vi "Query.vi"(8 "error in (no error)":errorcluster, 10 "command":string, 11 "Toolbox in":refnum<class "Toolbox.lvclass">) -> (0 "error out":errorcluster, 2 "responses":string[](array[string]), 3 "Toolbox out":refnum<class "Toolbox.lvclass">)   [LabVIEW 2014, in "Driver_interaction.lvlib" / "Toolbox.lvclass"]
uses:
  Toolbox.lvclass
  Toolbox.lvclass/Toolbox.ctl
  _Driver_interaction/_Driver_interaction.lvclass
  Vendor/lib 2p0/FTS 2p0.lvlib
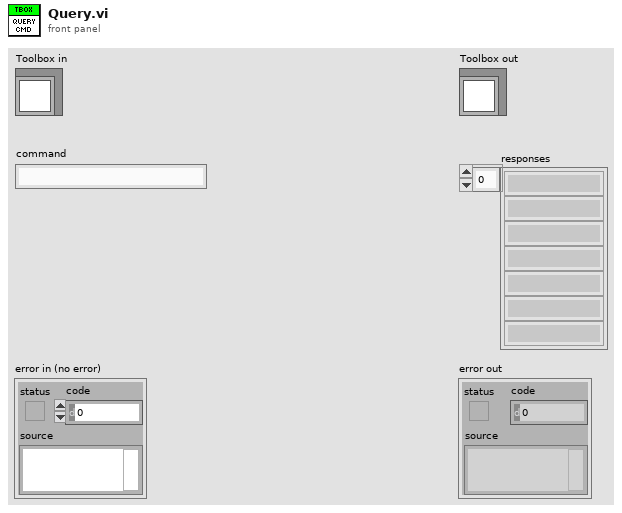
[diagram p1: front panel]
types:
  T1 = typedef "Driver_interaction.lvlib/Toolbox.lvclass/Toolbox_session.ctl" = cluster{"client handle":T2, "URL out":string, "universe_id":i32, "devices_id":i32[]}
  T2 = typedef "LabVIEWHTTPClient.lvlib/ClientHandle.ctl" = refnum<k1>
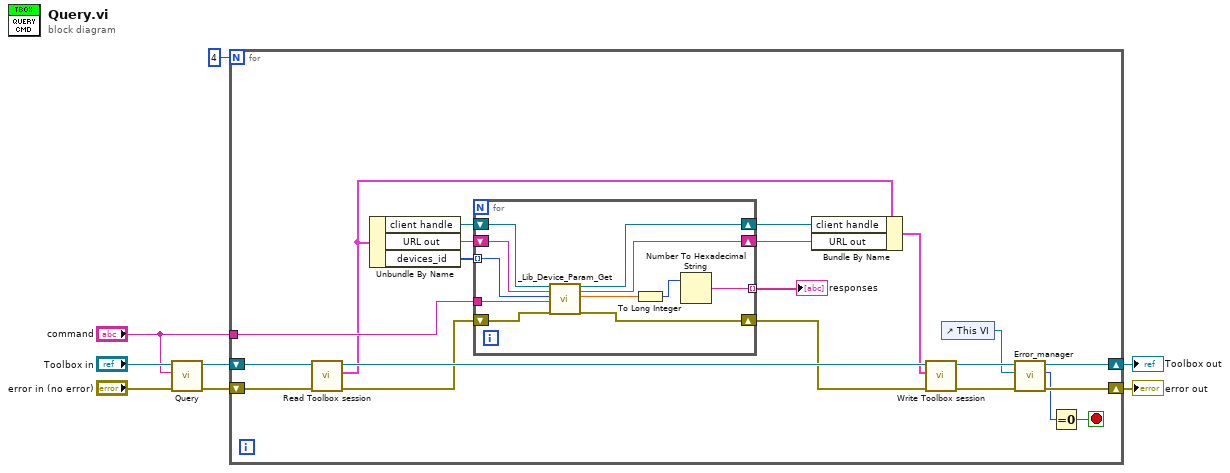
[diagram p0: block diagram]
diagram:
  n1 = call-parent "Query.vi"("error in (no error)"="error in (no error)", "command"="command", "_Driver_interaction in"="Toolbox in") -> ("error out"=w5:errorcluster, "_Driver_interaction out"=w6:refnum<class "Toolbox.lvclass">)  [unwired: 6 in, 1 out]
  n2 = for {
    N: 4 -> [_]
    tunnel: "command" -> [w22]
    shift-right: [w13] -> w4
    shift-left: w6 -> [w29]
    shift-right: [w12] -> w3
    shift-left: w5 -> [w27]
    stop <- w9 stop-if-true
    n3 = call "Read Toolbox session.vi"("error in (no error)"=w27, "Toolbox in"=w29) -> ("error out"=w26:errorcluster, "Toolbox session"=w21:T1, "Toolbox out"=w28:refnum<class "Toolbox.lvclass">)  [unwired: 7 in]
    n4 = Unbundle By Name(w21) -> ("client handle"=w24:T2, "URL out"=w23:string, "devices_id"=w17:i32[])
    n5 = for {
      tunnel: w22 -> [w36]
      tunnel: [w30] -> w16 mode=indexing
      shift-right: [w39] -> w25
      shift-left: w26 -> [w40]
      shift-right: [w35] -> w20
      shift-left: w24 -> [w38]
      shift-right: [w34] -> w19
      shift-left: w23 -> [w37]
      tunnel: w17 -> [w33] mode=indexing
      n6 = call "_Lib_Device_Param_Get.vi"("client handle"=w38, "URL"=w37, "params.device_id"=w33, "params.pid"=w36, "error in (no error)"=w40) -> ("client handle out"=w35:T2, "URL out"=w34:string, "value"=w32:dbl, "error out"=w39:errorcluster)  [unwired: 11 in]
      n7 = To Long Integer(number=w32) -> (32bit integer=w31:i32)
      n8 = Number To Hexadecimal String(2:w31) -> (0:w30:string)  [unwired: 1 in]
    }
    "responses" <- w16
    n9 = Bundle By Name(cluster=w21, "client handle"=w20, "URL out"=w19) -> (w18:T1)
    n10 = call "Write Toolbox session.vi"("error in (no error)"=w25, "Toolbox session"=w18, "Toolbox in"=w28) -> ("error out"=w15:errorcluster, "Toolbox out"=w14:refnum<class "Toolbox.lvclass">)  [unwired: 7 in]
    n11 = control-ref of="This VI"() -> (w11:refnum<vi>)
    n12 = call-dynamic "Error_manager.vi"("error in (no error)"=w15, "Caller VI"=w11, "Toolbox in"=w14) -> ("error out"=w12:errorcluster, "code"=w10:i32, "Toolbox out"=w13:refnum<class "Toolbox.lvclass">)  [unwired: 4 in, 2 out]
    n13 = Equal To 0?(x=w10) -> (x = 0?=w9:bool)
  }
  "error out" <- w3
  "Toolbox out" <- w4
